vi "Get I32.vi"(8 "error in (no error)":errorcluster, 11 "I32Message in":refnum<class "I32Message.lvclass">) -> (0 "error out":errorcluster, 2 "Message Data":i32, 3 "I32Message out":refnum<class "I32Message.lvclass">)   [LabVIEW 2009, in "LapDog.Messaging.v2.NativeTypes.lvlib" / "I32Message.lvclass"]
doc: "Returns the data contained in the message.\n\nThis method executes regardless of the error in state."
uses:
  I32Message.lvclass
  I32Message.lvclass/I32Message.ctl
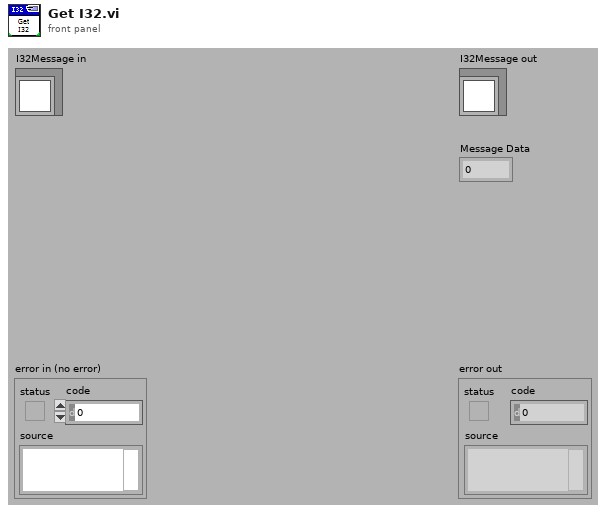
[diagram p1: front panel]
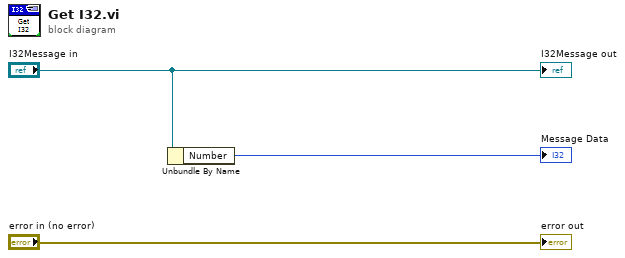
[diagram p0: block diagram]
diagram:
  n1 = Unbundle By Name("I32Message in") -> ("Number"=→"Message Data":i32)
  "error out" <- "error in (no error)"
  "I32Message out" <- "I32Message in"
